vi "FGV_Pockels Calibration.vi"(8 "error in (no error)":errorcluster, 9 "Function":T3=enum."Read", 10 "Pockels Cal table (Single wavelength)":string[][](array[string])) -> (0 "error out":errorcluster, 1 "Cal subset indexes":T2={"Start point index"=0, "End point index"=11}, 2 "Pockels calibration data (Single wavelength)":dbl[][](array[numeric]), 3 "Pockels cal header strings":string[](array[string]), 4 "Cal conditions":T1, 5 "Updated existing file?":bool, 7 "Multiplier for power after the objective":dbl)   [LabVIEW 2017]
uses:
  Typedefs/Functional global standard states.ctl
  Pockels Cal/Typedefs/Pockels cal conditions cluster.ctl
  Typedefs/Read Write Enum.ctl
  Typedefs/Which path.ctl
  gl_Calibration globals.vi
  <userlib>/My Palettes.lib/Files & paths/Spreadsheet/Read From Spreadsheet File (string)-Mod.vi
panel:
  out "SINGLE CAL SET / Pockels Cal table (inc. headers & info)":string[][](array[string])
  out "Wavelength value":dbl
  # "<-----The file name is picked up internally when this control is left blank"
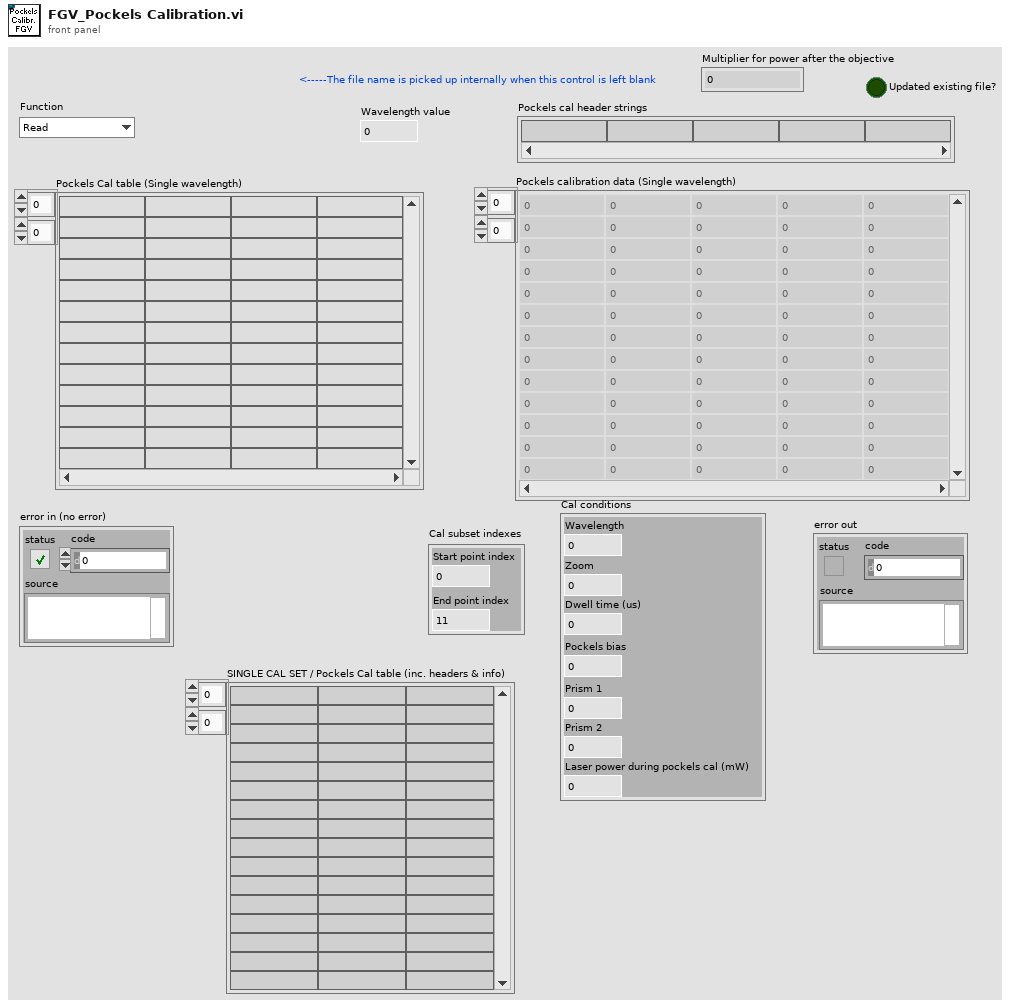
[diagram p1: front panel]
types:
  T1 = typedef "Pockels cal conditions cluster.ctl" = cluster{"Wavelength":u16, "Zoom":u8, "Dwell time (us)":dbl, "Pockels bias":i16, "Prism 1":u16, "Prism 2":u16, "Laser power during pockels cal (mW)":u16}
  T2 = cluster{"Start point index":i32, "End point index":i32}
  T3 = typedef "Functional global standard states.ctl" = enum16{"Initialise", "Read", "Write", "Load", "Save", "Clear"}
  T4 = typedef "Which path.ctl" = enum16{"Configuration Files", "Calibration Files", "Images", "Setup.ini", "Loaded User profile.ini", "User's-Previous session.ini", "New user profile.ini", "Selected User profile.ini", "User profiles folder", "Power meter scaling.txt", "FOV Cal.ini"}
  T5 = typedef "Read Write Enum.ctl" = enum16{"Read", "Write"}
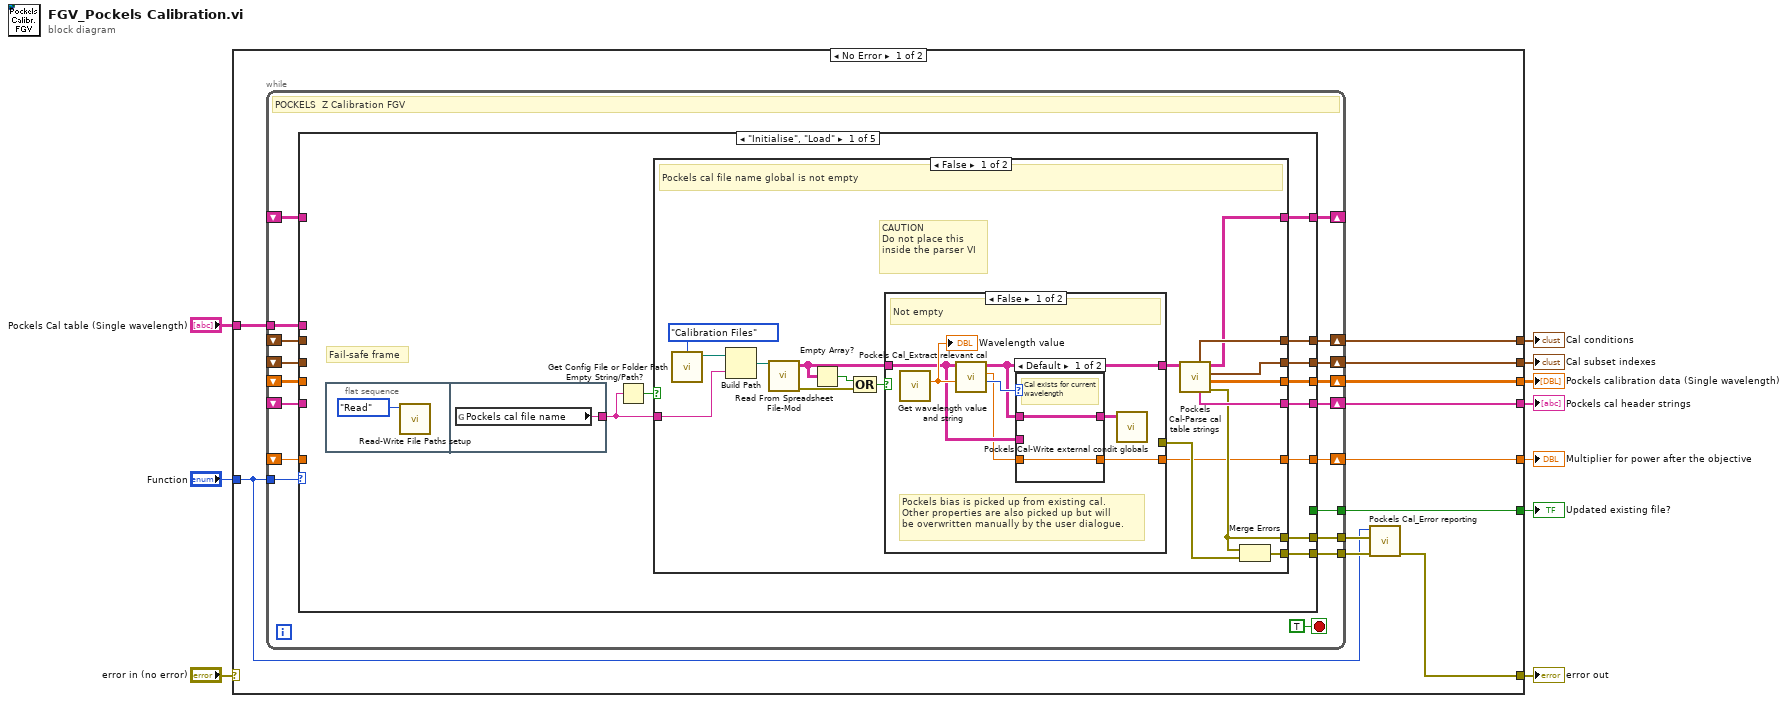
[diagram p0: block diagram]
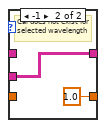
[diagram p2: hidden frame]
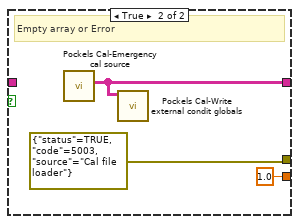
[diagram p3: hidden frame]
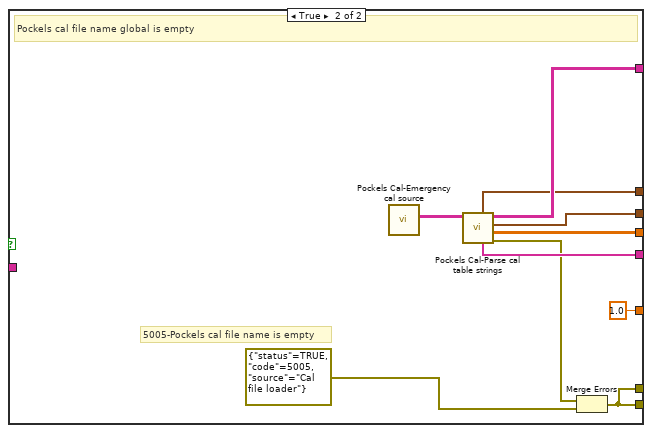
[diagram p4: hidden frame]
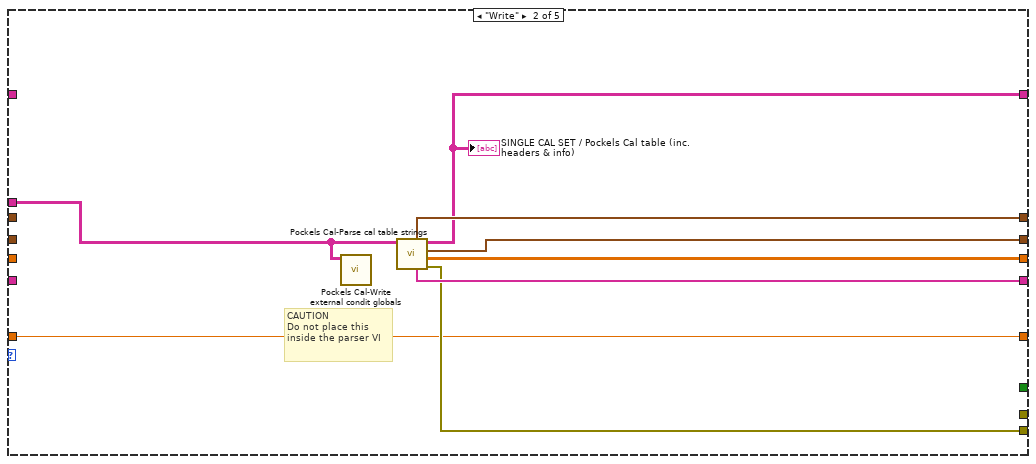
[diagram p5: hidden frame]
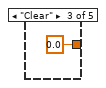
[diagram p6: hidden frame]
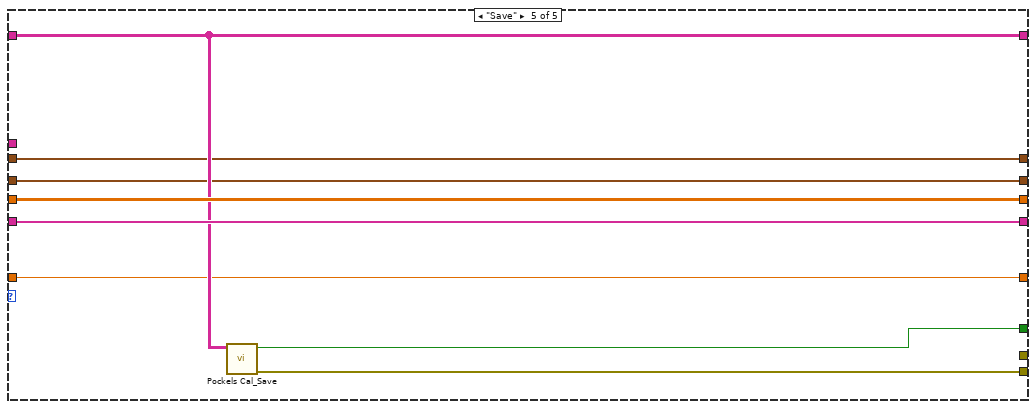
[diagram p8: hidden frame]
diagram:
  n1 = case shown="No Error" "error in (no error)" {
    selector: "error in (no error)" -> [_ w117]
    tunnel: [w13 w117] -> w6
    tunnel: "Function" -> [w15 _]
    tunnel: "Pockels Cal table (Single wavelength)" -> [w21 _]
    tunnel: [w20 _] -> w9
    tunnel: [w19 _] -> w8
    tunnel: [w17 _] -> w4
    tunnel: [w14 _] -> w3
    tunnel: [w12 _] -> w2
    tunnel: [w11 _] -> w1
    frame No Error {
      n2 = while {
        tunnel: w15 -> [w39]
        tunnel: w21 -> [w37]
        shift-right: [w36] -> w20
        shift-left: _ -> [w35]
        shift-right: [w34] -> w19
        shift-left: _ -> [w33]
        tunnel: [w28] -> w18
        shift-right: [w32] -> _
        shift-left: _ -> [w31]
        shift-right: [w30] -> w17
        shift-left: _ -> [w29]
        tunnel: [w27] -> w16
        shift-right: [w26] -> w14
        shift-left: _ -> [w25]
        tunnel: [w24] -> w12
        shift-right: [w22] -> w11
        shift-left: _ -> [w23]
        stop <- TRUE stop-if-true
        # "POCKELS  Z Calibration FGV"
        n3 = case shown="\"Initialise\", \"Load\"" w39 {
          tunnel: w37 -> [_ w96 _ _ _]
          tunnel: [w49 w101 _ w108 w116] -> w36
          tunnel: w35 -> [_ _ _ w108 w116]
          tunnel: [w48 w99 _ w107 w114] -> w34
          tunnel: w33 -> [_ _ _ w107 w114]
          tunnel: [w45 w95 _ w106 w113] -> w32
          tunnel: w31 -> [_ _ _ w106 w113]
          tunnel: [w44 w100 _ w105 w112] -> w30
          tunnel: w29 -> [_ _ _ w105 w112]
          tunnel: [w46 w98 _ _ w115] -> w28
          tunnel: [w43 _ _ _ _] -> w27
          tunnel: [w42 w97 _ w104 w111] -> w26
          tunnel: w25 -> [_ _ _ w104 w111]
          tunnel: [_ _ _ _ w110] -> w24
          tunnel: w23 -> [_ w94 _ w103 w109]
          tunnel: [w40 w94 0.0 ("Multiplier for power after the objective") w103 w109] -> w22
          frame "Initialise", "Load" {
            # "Fail-safe frame"
            n4 = flat-sequence {
              tunnel: [w93] -> w41
              frame #0 {
                n5 = call "Read-Write File Paths setup.vi"("Function"=Read_Write_Enum."Read") -> ()  [unwired: 10 in, 1 out]
              }
              frame #1 {
                n6 = global read "gl_Calibration globals.vi" "Pockels cal file name"() -> (w93:string)
              }
            }
            n7 = Empty String/Path?(string/path=w41) -> (empty?=w47:bool)
            n8 = case shown="False" w47 {
              tunnel: [w61 w90] -> w49
              tunnel: [w59 w88] -> w48
              tunnel: w41 -> [w65 _]
              tunnel: [w58 w86] -> w46
              tunnel: [w51 w91] -> w45
              tunnel: [w60 w89] -> w44
              tunnel: [w57 w86] -> w43
              tunnel: [w56 w85] -> w42
              tunnel: [w50 1.0 ("Multiplier for power after the objective")] -> w40
              frame False {
                # "CAUTION\nDo not place this  inside the parser VI"
                # "Pockels cal file name global is not empty"
                n9 = call "Get Config File or Folder Path.vi"("Which file or folder?"=Which_path."Calibration Files" ("Which path?")) -> ("File Path"=w66:path)  [unwired: 8 in, 2 out]
                n10 = Build Path(base path=w66, name or relative path=w65) -> (appended path=w64:path)
                n11 = call-poly <userlib>:"Read From Spreadsheet File-Mod.vi"("file path (dialog if empty)"=w64) -> ("all rows"=w55:string[][], "error out"=w53:errorcluster)  [unwired: 9 in, 4 out]
                n12 = Empty Array?(array=w55) -> (empty?=w63:bool)
                n13 = Compound Arithmetic op=OR(w63, w53) -> (w62:bool)
                n14 = case shown="False" w62 {
                  tunnel: w55 -> [w70 _]
                  tunnel: [w72 w80] -> w54
                  tunnel: [_ errorcluster {"status"=TRUE, "code"=5003, "source"="Cal file loader"} ("error out")] -> w52
                  tunnel: [w69 1.0 ("Multiplier for power after the objective")] -> w50
                  frame False {
                    # "Pockels bias is picked up from existing cal.\nOther properties are also picked up but will\nbe overwritten manually by the user dialogue."
                    # "Not empty"
                    n15 = call "Get wavelength value and string.vi"() -> ("Wavelength value"=w74:dbl)  [unwired: 9 in, 2 out]
                    "Wavelength value" <- w74
                    n16 = call "Pockels Cal_Extract relevant cal.vi"("Wavelength value"=w74, "Loaded table"=w70) -> ("Index of replacement"=w73:i32, "Multiplier for power after the objective"=w68:dbl, "Relevant cal only"=w72:string[][])  [unwired: 6 in, 1 out]
                    n17 = case shown="Default" w73 {
                      tunnel: w72 -> [w76 _]
                      tunnel: [w76 w78] -> w71
                      tunnel: w70 -> [_ w78]
                      tunnel: [w75 1.0] -> w69
                      tunnel: w68 -> [w75 _]
                      frame Default {
                        # "Cal exists for current wavelength"
                      }
                      frame -1 {
                        # "Cal does not exist for selected wavelength"
                      }
                    }
                    n18 = call "Pockels Cal-Write external condit globals.vi"("Pockels Cal table"=w71) -> ()  [unwired: 11 in]
                  }
                  frame True {
                    # "Empty array or Error"
                    n19 = call "Pockels Cal-Emergency cal source.vi"() -> ("SINGLE CAL SET (inc. headers & info)"=w80:string[][])  [unwired: 11 in]
                    n20 = call "Pockels Cal-Write external condit globals.vi"("Pockels Cal table"=w80) -> ()  [unwired: 11 in]
                  }
                }
                n21 = call "Pockels Cal-Parse cal table strings.vi"("SINGLE CAL SET (inc. headers & info)"=w54) -> ("error out"=w57:errorcluster, "Pockels Cal data"=w61:dbl[][], "Cal subset indexes"=w60:T2, "SINGLE CAL SET / Pockels Cal table (inc. headers & info)"=w51:string[][], "Cal data header"=w59:string[], "Cal conditions"=w56:T1)  [unwired: 5 in]
                n22 = Merge Errors(w57, w52) -> (w58:errorcluster)
              }
              frame True {
                # "5005-Pockels cal file name is empty"
                # "Pockels cal file name global is empty"
                n23 = call "Pockels Cal-Emergency cal source.vi"() -> ("SINGLE CAL SET (inc. headers & info)"=w84:string[][])  [unwired: 11 in]
                n24 = call "Pockels Cal-Parse cal table strings.vi"("SINGLE CAL SET (inc. headers & info)"=w84) -> ("error out"=w87:errorcluster, "Pockels Cal data"=w90:dbl[][], "Cal subset indexes"=w89:T2, "SINGLE CAL SET / Pockels Cal table (inc. headers & info)"=w91:string[][], "Cal data header"=w88:string[], "Cal conditions"=w85:T1)  [unwired: 5 in]
                n25 = Merge Errors(w87, errorcluster {"status"=TRUE, "code"=5005, "source"="Cal file loader"} ("error out")) -> (w86:errorcluster)
              }
            }
          }
          frame "Write" {
            # "CAUTION\nDo not place this  inside the parser VI"
            n26 = call "Pockels Cal-Write external condit globals.vi"("Pockels Cal table"=w96) -> ()  [unwired: 11 in]
            n27 = call "Pockels Cal-Parse cal table strings.vi"("SINGLE CAL SET (inc. headers & info)"=w96) -> ("error out"=w98:errorcluster, "Pockels Cal data"=w101:dbl[][], "Cal subset indexes"=w100:T2, "SINGLE CAL SET / Pockels Cal table (inc. headers & info)"=w95:string[][], "Cal data header"=w99:string[], "Cal conditions"=w97:T1)  [unwired: 5 in]
            "SINGLE CAL SET / Pockels Cal table (inc. headers & info)" <- w95
          }
          frame "Clear" {
          }
          frame "Read", Default {
          }
          frame "Save" {
            n28 = call "Pockels Cal_Save.vi"("Pockels Cal table (inc. headers & info)"=w113) -> ("error out"=w115:errorcluster, "Updated existing file?"=w110:bool)  [unwired: 9 in]
          }
        }
      }
      n29 = call "Pockels Cal_Error reporting.vi"("error in (no error)"=w18, "error IO"=w16, "Function"=w15) -> ("error out"=w13:errorcluster)  [unwired: 8 in]
    }
    frame Error {
    }
  }
  "error out" <- w6
  "Pockels calibration data (Single wavelength)" <- w9
  "Pockels cal header strings" <- w8
  "Cal subset indexes" <- w4
  "Cal conditions" <- w3
  "Updated existing file?" <- w2
  "Multiplier for power after the objective" <- w1
